vi "SMC_SetVel.vi"(8 "error in (no error)":errorcluster, 11 "Velocity":dbl format="%.3f") -> (0 "error out":errorcluster)   [LabVIEW 2015]
uses:
  SMC_SubVIs.llb/SMC_ManagerMode.ctl
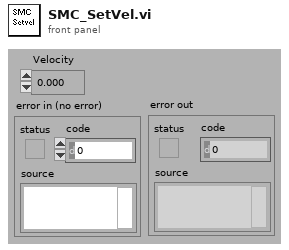
[diagram p1: front panel]
types:
  T1 = typedef "SMC_ManagerMode.ctl" = enum16{"Init", "Get", "SetPosition", "SetStatus", "SetMoving", "SetControllerNr"}
  T2 = typedef "SMC Paras.ctl" = cluster{"VENUS Language":T3, "Number of Axis":u8, "Controller Nr":u8, "Simulation":bool}
  T3 = typedef "VENUSNr.ctl" = enum16{"VENUS 2", "VENUS 1"}
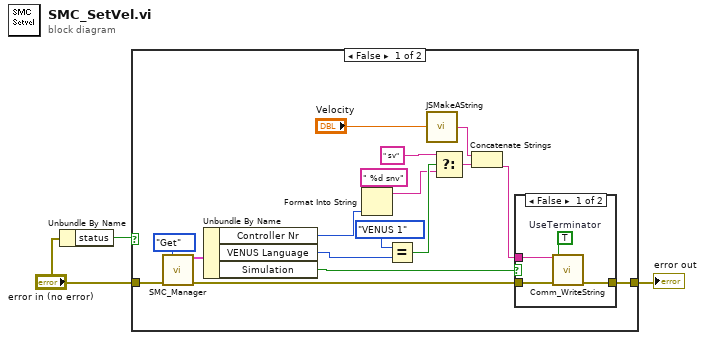
[diagram p0: block diagram]
diagram:
  n1 = Unbundle By Name("error in (no error)") -> ("status"=w3:bool)
  n2 = case shown="False" w3 {
    tunnel: "error in (no error)" -> [w20 w26]
    tunnel: [w17 w26] -> w1
    frame False {
      n3 = call "SMC_Manager.vi"("Mode"=SMC_ManagerMode."Get", "error in (no error)"=w20) -> ("SMC Parameter Out"=w7:T2, "error out"=w18:errorcluster)  [unwired: 9 in, 3 out]
      n4 = Unbundle By Name(w7) -> ("Controller Nr"=w5:u8, "VENUS Language"=w6:T3, "Simulation"=w4:bool)
      n5 = Format Into String(format string=" %d snv" ("Format String"), w5) -> (resulting string=w13:string)  [unwired: 2 in, 1 out]
      n6 = Equal?(x=enum16{"VENUS 2", "VENUS 1"}."VENUS 1", y=w6) -> (x = y?=w14:bool)
      n7 = call "JSMakeAString.vi"("Value"="Velocity") -> ("String"=w9:string)
      n8 = Select(t=" sv" ("Format String"), s=w14, f=w13) -> (s? t:f=w10:string)
      n9 = Concatenate Strings(w9, w10) -> (w8:string)
      n10 = case shown="False" w4 {
        tunnel: w8 -> [w24 _]
        tunnel: w18 -> [w23 w25]
        tunnel: [w22 w25] -> w17
        frame False {
          w21 = TRUE  # UseTerminator
          n11 = call "Comm_WriteString.vi"("string to write"=w24, "error in (no error)"=w23, "UseTerminator"=w21) -> ("error out"=w22:errorcluster)  [unwired: 8 in]
        }
        frame True {
          # "Simulation"
        }
      }
    }
    frame True {
      # "Error, do nothing"
    }
  }
  "error out" <- w1
